vi "UMLEditor_RelativePath.vi"(0 "Path In":path, 2 "error in (no error)":errorcluster) -> (10 "ConvertedToARelativePath":bool, 12 "ConvertToRelativePath(If possible)":path, 14 "ConvertToAbsolutePath(If possible)":path, 15 "ConvertedToAbsolutePath":bool, 16 "error out":errorcluster)   [LabVIEW 2016]
uses:
  <resource>/Framework/Providers/Open_GDS/UML/UMLEditor/UMLEditor_StoredPathes.ctl
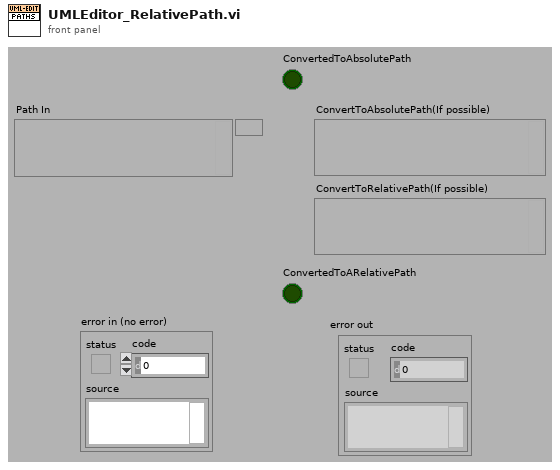
[diagram p1: front panel]
types:
  T1 = typedef "UMLEditor_StoredPathes.ctl" = enum16{"LastSearchPath", "QueuedArrayStateVI", "ClassBasePath", "ViTemplatePath", "ApplicationTemplatePath", "IniFilePath", "WizDir", "RevPlugInPath"}
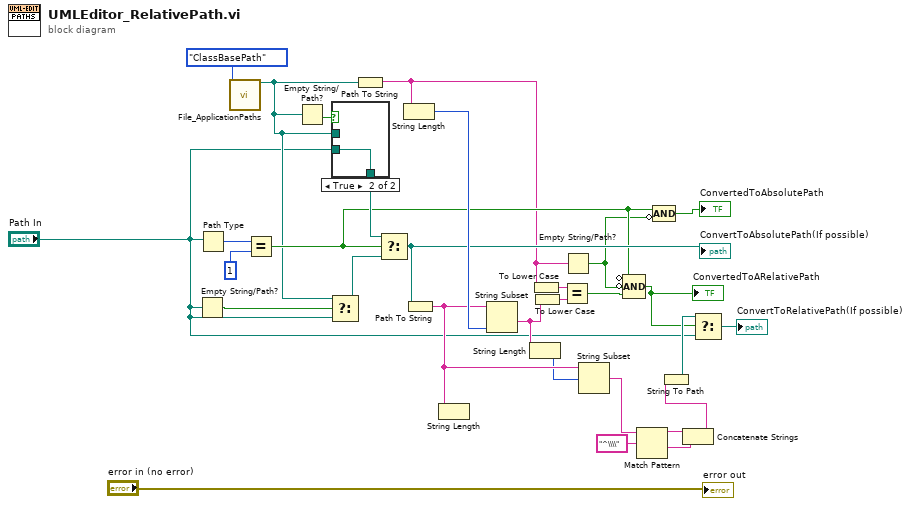
[diagram p0: block diagram]
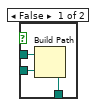
[diagram p2: hidden frame]
diagram:
  n1 = Empty String/Path?(string/path="Path In") -> (empty?=w10:bool)
  n2 = Path Type(1:"Path In") -> (0:w28:i16)
  n3 = call <resource>:"File_ApplicationPaths.vi"("PathName"=UMLEditor_StoredPathes."ClassBasePath" ("UMLPathes")) -> ("Path Out"=w5:path)  [unwired: 3 in, 15 out]
  n4 = Equal?(x=w28, y=i16 1) -> (x = y?=w7:bool)
  n5 = Empty String/Path?(string/path=w5) -> (empty?=w4:bool)
  n6 = Select(t=w5, s=w10, f="Path In") -> (s? t:f=w9:path)
  n7 = case shown="True" w4 {
    tunnel: [w33 w34] -> w26
    tunnel: "Path In" -> [w32 w34]
    tunnel: w5 -> [w31 _]
    frame False {
      n8 = Build Path(base path=w31, name or relative path=w32) -> (appended path=w33:path)
    }
    frame True {
    }
  }
  n9 = Path To String(path=w5) -> (string=w6:string)
  n10 = Select(t=w26, s=w7, f=w9) -> (s? t:f=w11:path)
  "ConvertToAbsolutePath(If possible)" <- w11
  n11 = String Length(string=w6) -> (length=w25:i32)
  n12 = Path To String(path=w11) -> (string=w22:string)
  n13 = String Length(string=w22) -> ()  [unwired: 1 out]
  n14 = String Subset(string=w22, length (rest)=w25) -> (substring=w21:string)  [unwired: 1 out]
  n15 = String Length(string=w21) -> (length=w20:i32)
  n16 = To Lower Case(string=w6) -> (all lower case string=w24:string)
  n17 = To Lower Case(string=w21) -> (all lower case string=w23:string)
  n18 = Equal?(x=w24, y=w23) -> (x = y?=w14:bool)
  n19 = Empty String/Path?(string/path=w6) -> (empty?=w2:bool)
  n20 = String Subset(string=w22, offset (0)=w20) -> (substring=w18:string)  [unwired: 1 out]
  n21 = Compound Arithmetic op=AND(invert w7, invert w2, w14) -> (w8:bool)
  "ConvertedToARelativePath" <- w8
  n22 = Match Pattern(string=w18, regular expression="^\\\\") -> (before substring=w17:string, after substring=w16:string)  [unwired: 3 out]
  n23 = Compound Arithmetic op=AND(w7, invert w2) -> (→"ConvertedToAbsolutePath":bool)
  n24 = Concatenate Strings(w17, w16) -> (w15:string)
  n25 = String To Path(string=w15) -> (path=w13:path)
  n26 = Select(t=w13, s=w8, f="Path In") -> (s? t:f=→"ConvertToRelativePath(If possible)":path)
  "error out" <- "error in (no error)"
